vi "Fdx Set Call Library Path.vi"() -> (3 "DllPath":path=path "aim_fdx.19.dll")   [LabVIEW 2020, in "AIM664LV.lvlib"]
uses:
  AIM664LV.lvlib
  AFDX_LibraryAdmin/FdxGlobalDllPath.vi
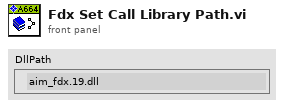
[diagram p1: front panel]
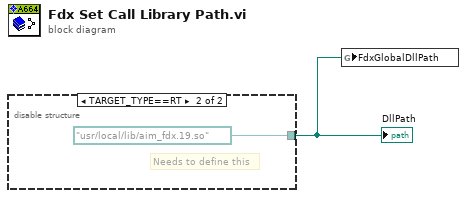
[diagram p0: block diagram]
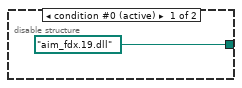
[diagram p2: hidden frame]
diagram:
  n1 = disable-structure "Conditional Disable Structure" shown="TARGET_TYPE==RT" {
    disable-tunnel: [path "aim_fdx.19.dll" ("GlobalDLLPath") path "/usr/local/lib/aim_fdx.19.so" ("DLL Path (if required)")] -> w1
    frame condition #0 (active) {
    }
    frame condition #1 {
      # "Needs to define this"
    }
  }
  "DllPath" <- w1
  n2 = global write "FdxGlobalDllPath.vi" "FdxGlobalDllPath"(w1) -> ()
